vi "SI5 FPGA.vi"() -> ()   [LabVIEW 2014]
uses:
  Acquisition Engine/Acquisition Engine State.ctl
  Adapter Module Specific/Multi-Channel Analog Input Data.ctl
  <vilib>/Platform/TimedLoop/XDataNode/timing_clust.ctl
  <vilib>/Platform/TimedLoop/XDataNode/nitl_modes.ctl
  <vilib>/Platform/TimedLoop/XDataNode/wakeup.ctl
  Acquisition Engine/Acquisition Parameters.ctl
  Adapter Module Specific/Trigger Type.ctl
  <vilib>/rvi/Emulation/niFpgaSctlEmulationGetInTimedLoop.vi
  <vilib>/rvi/Emulation/niFpgaProcessEmulError.vi
  <vilib>/rvi/Emulation/niFpgaEmulationReportErrorSimple.vi
  <vilib>/rvi/Emulation/niFpgaGetClockAttributes.vi
  <vilib>/rvi/Emulation/niFpgaCriticalErrorInLSC.vi
  <vilib>/rvi/eio/common/nirviEmuTemplateMethod_errors.vi
  <vilib>/rvi/DataTransferAndStorage/Container/Common/niFpgaContainerGetUniqueNameForEmu.vi
  <vilib>/rvi/DataTransferAndStorage/Container/Common/niFpgaContainerSetEmuInfo.vi
  <vilib>/rvi/eio/common/nirviEmuReportErrorAndStop.vi
  <vilib>/rvi/DataTransferAndStorage/Container/Common/niFpgaContainerExecOnDevCompGetState.vi
  <vilib>/rvi/Emulation/niFpgaEmulationIsFPGAContextNoSignature.vi
  <vilib>/rvi/errors/niFpgaSetErrorForExecOnDevCompSimple.vi
  <vilib>/rvi/FIFO/Fifo_Resource/nirvififoEmulationSetSize.vi
  <vilib>/rvi/FIFO/Fifo_Resource/nirviFifoEmulationQueueMgr.vi
  <instcachedir>/0/nirviFifoEmulationQueueMgr_E5CAEC123FF24DC58D834DCA3CDAA9B5.lvgen/nirviFifoEmulationQueueMgr_E5CAEC123FF24DC58D834DCA3CDAA9B5_001.vi
  <vilib>/rvi/FIFO/Fifo_Resource/nirvififoEmulationDetermineInputValidOut.vi
  <vilib>/rvi/FIFO/Fifo_Resource/nirvififoEmulationCreateLock.vi
  <vilib>/rvi/FIFO/Fifo_Resource/nirvififoEmulationObtainLock.vi
  <vilib>/rvi/FIFO/Fifo_Resource/nirvififoEmulationReleaseLock.vi
  <vilib>/rvi/occurrence/nirviWaitOnOccurrenceBase.vi
  <vilib>/rvi/errors/nirviReportUnexpectedCaseInternalError.vi
  <vilib>/rvi/errors/nirviReportUnexpectedCaseInternalError (U32).vi
  <vilib>/rvi/interface/RandomDataEmulation/niFpgaRandomDataHandleErrors.vi
  <vilib>/Platform/TimedLoop/XDataNode/XDataNode.xnode
  <vilib>/eio/EIONode/EIONode.xnode
  <vilib>/rvi/LocalResourceManager/LocalResourceManager.xnode
  <vilib>/rvi/DataTransferAndStorage/Container/XNode/niFpgaContainer.xnode
  <vilib>/rvi/FIFO/Fifo_Resource/niFpgaFifoEmulationRefIn.vi
  <vilib>/Platform/TimedLoop/XDataNode/XDNodeRunTimeDep.lvlib
panel:
  in  "SPI Read":bool caption="(Mech Action: Switch)"
  in  "SPI Write":bool caption="(Mech Action: Switch)"
  in  "SPI Write Data":u16
  in  "SPI Address":u16
  in  "SPI Device Select":u8
  out "SPI Read Data":u8
  out "SPI Idle":bool
  in  "Acq Param Frames Per Stack":u16
  in  "Shutter Output":bool
  in  "Shutter Terminal Out":T1(ring)=enum.""
  out "Acq Status DC Overvoltage":bool
  in  "Acq Param Live Invert Channels":bool
  out "Acq Status Acquired Grabs":u16
  in  "Period Clock Terminal Out":T1(ring)=enum.""
  in  "Acq Trigger Terminal Out 2":T1(ring)=enum.""
  in  "Beam Clock Terminal Out 2":T1(ring)=enum.""
  in  "Frame Clock Terminal Out 2":T1(ring)=enum.""
  in  "Acq Trigger Terminal Out":T1(ring)=enum.""
  out "Debug Raw Adc Output":T2
  in  "Acq Param Live Channel Offsets":T2=[0, 0, 0, 0]
  in  "Irq Number Fifo Multi Channel Pixel Overwritten By Tag":i8=-1
  in  "Irq Number Fifo Single Channel Pixel Overwritten By Tag":i8=-1
  in  "Irq Number End of Acquisition":i8=-1
  in  "Irq Number End of Grab":i8=-1
  in  "Acq Param Grabs Per Acquisition":u16
  in  "Beam Clock Off Backward":i16
  in  "Beam Clock On Backward":i16
  in  "Beam Clock Off Forward":i16
  in  "Beam Clock On Forward":i16
  in  "Beam Clock Mode":enum8{"Trigger", "Toggle"}(ring)=enum."Toggle"
  in  "Beam Clock Terminal Out":T1(ring)=enum.""
  in  "Frame Clock Terminal Out":T1(ring)=enum.""
  in  "Stop Trigger Do Software Trig":bool
  in  "Stop Trigger Type":T3(ring)=enum."External or Software"
  in  "Stop Trigger On Falling Edge":bool
  in  "Advance Trigger Do Software Trig":bool
  in  "Advance Trigger Type":T3(ring)=enum."External or Software"
  in  "Advance Trigger On Falling Edge":bool
  in  "Stop Trigger Terminal In":T4(ring)=enum.""
  in  "Advance Trigger Terminal In":T4(ring)=enum.""
  out "Acq Status Acquired Frames":u32
  in  "Acq Param Flyback Periods":u8
  in  "Acq Param Records Per Frame":u16
  out "Adapter Module Present":bool
  in  "Acq Param Live Reverse Line Read":bool
  out "Adapter Module ID Expected":u32
  out "Adapter Module ID Inserted":u32
  in  "Acq Param Frame Tagging Enable":bool
  in  "Acq Trigger On Falling Edge":bool
  in  "Acq Trigger Type":T3(ring)=enum."External or Software"
  in  "Acq Trigger Do Software Trig":bool
  in  "Acq Trigger Terminal In":T4(ring)=enum.""
  in  "Debug Produce Dummy Data":bool
  out "Adapter Module Initialization Done":bool
  in  "Irq Number Fifo Single Channel Overflow":i8=-1
  in  "Irq Number Fifo Multi Channel Overflow":i8=-1
  in  "Irq Number End of Frame":i8=-1
  in  "Irq Fifos Data Lost Do Rearm":bool caption="(Mech Action: Latch)"
  out "Fifo Multi Channel Pixels Lost":u32
  out "Fifo Single Channel Pixels Lost":u32
  in  "Fifo Enable Multi Channel":bool
  in  "Fifo Enable Single Channel":bool
  in  "Period Clock Terminal In":T4(ring)=enum.""
  out "Adapter Module ID Mismatch":bool
  in  "Acq Param Frames Per Grab":u32 caption="Record Count"
  in  "Acq Param Live Trigger Hold Off":u16
  in  "Acq Param Samples Per Record":u16
  in  "Acq Param Live Pre Trigger Samples":u16
  in  "Period Clock On Falling Edge":bool
  out "Acq Status Acquired Records":u32
  in  "Debug Disable Raster Flip":bool
  in  "Mask Do Write Element":bool caption="(Mech Action: Latch)"
  in  "Mask Element Data":i16
  in  "Mask Write Index":i32
  out "Acq Status Acquired Pixels":u64
  in  "Adapter Module Do User Command Commit":bool caption="(Mech Action: Latch)"
  in  "Adapter Module User Command":u8
  out "Adapter Module User Command Idle":bool
  out "Adapter Module User Command Status":u8
  in  "Adapter Module User Data 0":u8
  in  "Adapter Module User Data 1":u8
  out "Adapter Module PLL Locked":bool
  in  "Acq Engine Do Reset":bool caption="(Mech Action: Latch)"
  in  "Acq Engine Do Arm":bool caption="(Mech Action: Latch)"
  in  "Period Clock Do Software Trig":bool
  in  "Acq Param Live Select Single Channel":T5(ring)
  out "Acq Status Acquired Adc Samples":u64
  out "Acq Status Engine State":T6
  in  "Period Clock Type":T3(ring)=enum."External or Software"
  # "Copyright 2014 Vidrio Technologies\nScanImage 5 software is licensed under the Apache License, Version 2.0 (the \"License\"); you may not use any files contained within the ScanImage 5 release except in compliance with the License. You may obtain a copy of the License at\n http://www.apache.org/licenses/LICENSE-2.0\nUnless required by applicable law or agreed to in writing, software distributed under the License is distributed on an \"AS IS\" BASIS, WITHOUT WARRANTIES OR CONDITIONS OF ANY KIND, either express or implied. See the License for the specific language governing permissions and limitations under the License."
  # "Acquisition Parameters"
  # "Acquisition Control"
  # "User Command Load"
  # "Fpga status"
  # "Beam Clock"
  # "SPI"
  # "Mask"
  # "Acquisition Status & Debug"
  # "Trigger I"
  # "Trigger II"
  # "Trigger III"
  # "Interrupts"
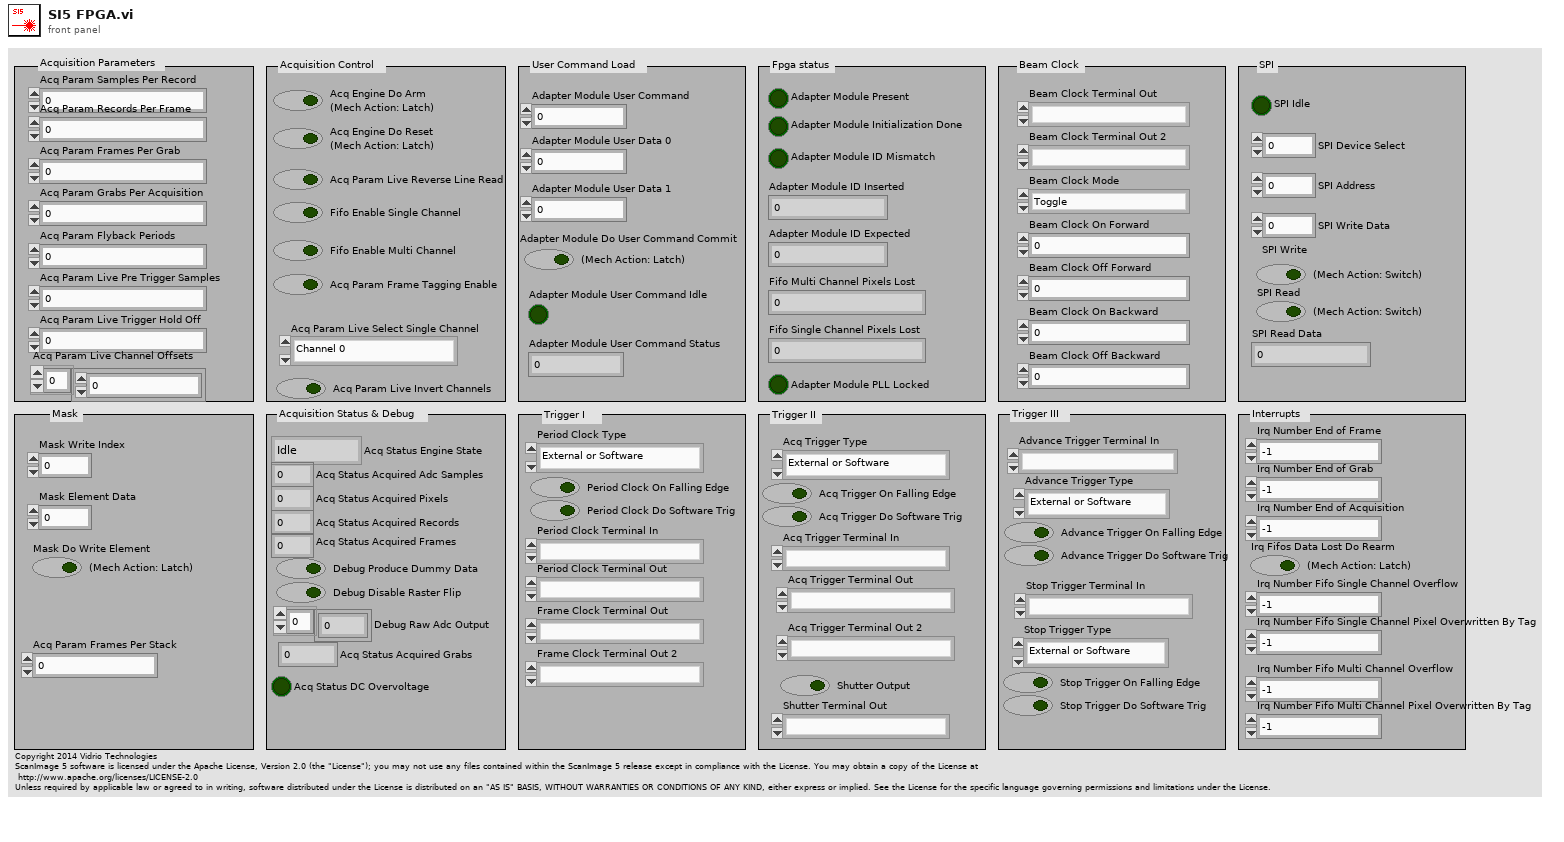
[diagram p1: front panel]
types:
  T1 = enum8{"DIO1.0", "DIO1.1", "DIO1.2", "DIO1.3", "PXI_Trig0", "PXI_Trig1", "PXI_Trig2", "PXI_Trig3", "PXI_Trig4", "PXI_Trig5", "PXI_Trig6", "PXI_Trig7", ""}
  T2 = typedef "Multi-Channel Analog Input Data.ctl" = i16[]
  T3 = enum8{"External", "Software", "Immediate", "External or Software", "None"}
  T4 = enum8{"DIO0.0", "DIO0.1", "DIO0.2", "DIO0.3", "PXI_Trig0", "PXI_Trig1", "PXI_Trig2", "PXI_Trig3", "PXI_Trig4", "PXI_Trig5", "PXI_Trig6", "PXI_Trig7", ""}
  T5 = enum8{"Channel 0", "Channel 1", "Channel 2", "Channel 3"}
  T6 = typedef "Acquisition Engine State.ctl" = enum8{"Idle", "Wait for Trigger", "Acquisition Hold Off Time", "Read Data", "Check Frame Done", "Check Grab Done", "Check Acquisition Done", "Wait Flyback Periods", "Flush Data"}
  T7 = typedef "XDNodeRunTimeDep.lvlib/timing_clust.ctl" = cluster{"Expected End [f-1]":u64, "Actual End [f-1]":u64, "Finished Late? [f-1]":bool, "Expected End [i-1]":u64, "Actual End [i-1]":u64, "Finished Late? [i-1]":bool, "Expected Start [i]":u64, "Actual Start [i]":u64, "Expected Start [f]":u64, "Actual Start [f]":u64, "Source Name":string, "Structure Name":string, "Period":i64, "Deadline":i64, "Offset":i64, "Start":i64, "Priority":i32, "Timeout":i32, "Mode":T8, "Wakeup Reason":T9, "Error":errorcluster, "Source Type":string, "Secondary Source Type":string, "Global End Time":u64, "Global Start Time":u64, "Frame Duration":u64, "Iteration Duration":u64, "Assigned CPU":i32, "I/O Scan Engine Mode":u32}
  T8 = typedef "XDNodeRunTimeDep.lvlib/nitl_modes.ctl" = enum32{"No Change", "Process missed periods, maintain original phase", "Discard missed periods, maintain original phase", "Process missed periods, ignore original phase", "Discard missed periods, ignore original phase"}
  T9 = typedef "XDNodeRunTimeDep.lvlib/wakeup.ctl" = enum32{"Normal", "Aborted", "Asynchronous wakeup", "Timing source error", "Timed loop error", "Timeout"}
  T10 = typedef "Trigger Type.ctl" = enum8{"External", "Software", "Immediate", "External or Software", "None"}
  T11 = cluster{"Acq Trigger Type":T10, "Acq Trigger On Falling Edge":bool, "Acq Software Trigger from Host":bool, "Period Clock Type":T10, "Period Clock On Falling Edge":bool, "Period Software Trigger from Host":bool, "Advance Trigger Type":T10, "Advance Trigger On Falling Edge":bool, "Advance Software Trigger from Host":bool, "Stop Trigger Type":T10, "Stop Trigger On Falling Edge":bool, "Stop Software Trigger from Host":bool}
  T12 = cluster{"Acq Engine Do Arm":bool, "Acq Engine Do Reset":bool}
  T13 = typedef "Acquisition Parameters.ctl" = cluster{"Trigger Hold Off":u16, "Samples per Record":u16, "Records Per Frame":u16, "Frames Per Grab":u32, "Grabs Per Acquisition":u16, "Flyback Periods":u8, "Frames Per Stack":u16, "Beam Clock Config":cluster{"Beam Clock Mode":enum8{"Trigger", "Toggle"}, "Beam On Forward":i16, "Beam Off Forward":i16, "Beam On Backward":i16, "Beam Off Backward":i16}}
  T14 = cluster{"Rearm FIFO Data Lost IRQs":bool, "Enable FIFO Single Channel":bool, "Enable FIFO Multi Channel":bool}
  T15 = cluster{"Bank 0":refnum<k21>, "Bank 1":refnum<k21>}
  T16 = typedef "Trigger Signals.ctl" = cluster{"Acquisition Trigger":bool, "Period Clock":bool, "Advance Trigger":bool, "Stop Trigger":bool}
  T17 = typedef "Acquisition Status.ctl" = cluster{"Reset":bool, "Start of Record":bool, "End of Record":bool, "Start of Frame":bool, "End of Frame":bool, "End of Grab":bool, "End of Acquisition":bool, "Frame Timestamp":u64, "Acq Trigger Timestamp":u64, "Next Trigger Timestamp":u64}
  T18 = typedef "Trigger Output Signals.ctl" = cluster{"Period Clock":bool, "Frame Clock":bool, "Beam Clock":bool, "Acquisition Trigger":bool}
  T19 = cluster{"Acquisition State":T6, "Updated Grabs Done":u16}
  T20 = typedef "Async Frametag Data.ctl" = cluster{"Send Frametag":bool, "End Of Grab":bool, "End of Acquisition":bool, "Next Trigger Timestamp":u64}
  T21 = cluster{"Mask Write Index":i32, "Mask Element Data":i16, "Mask Do Write Element":bool}
  T22 = cluster{"EndofLine?":bool, "Acquisition Status Out":T17}
  T23 = cluster{"Single Channel Output":cluster{"Single Channel Data out":i16, "Output Valid":bool, "Pixel Overwritten by Tag":bool}, "Multi Channel Output":cluster{"Multi Channel Data out":i16[], "Output Valid":bool, "Pixel Overwritten by Tag":bool}}
  T24 = typedef "IRQ Flags.ctl" = bool[]
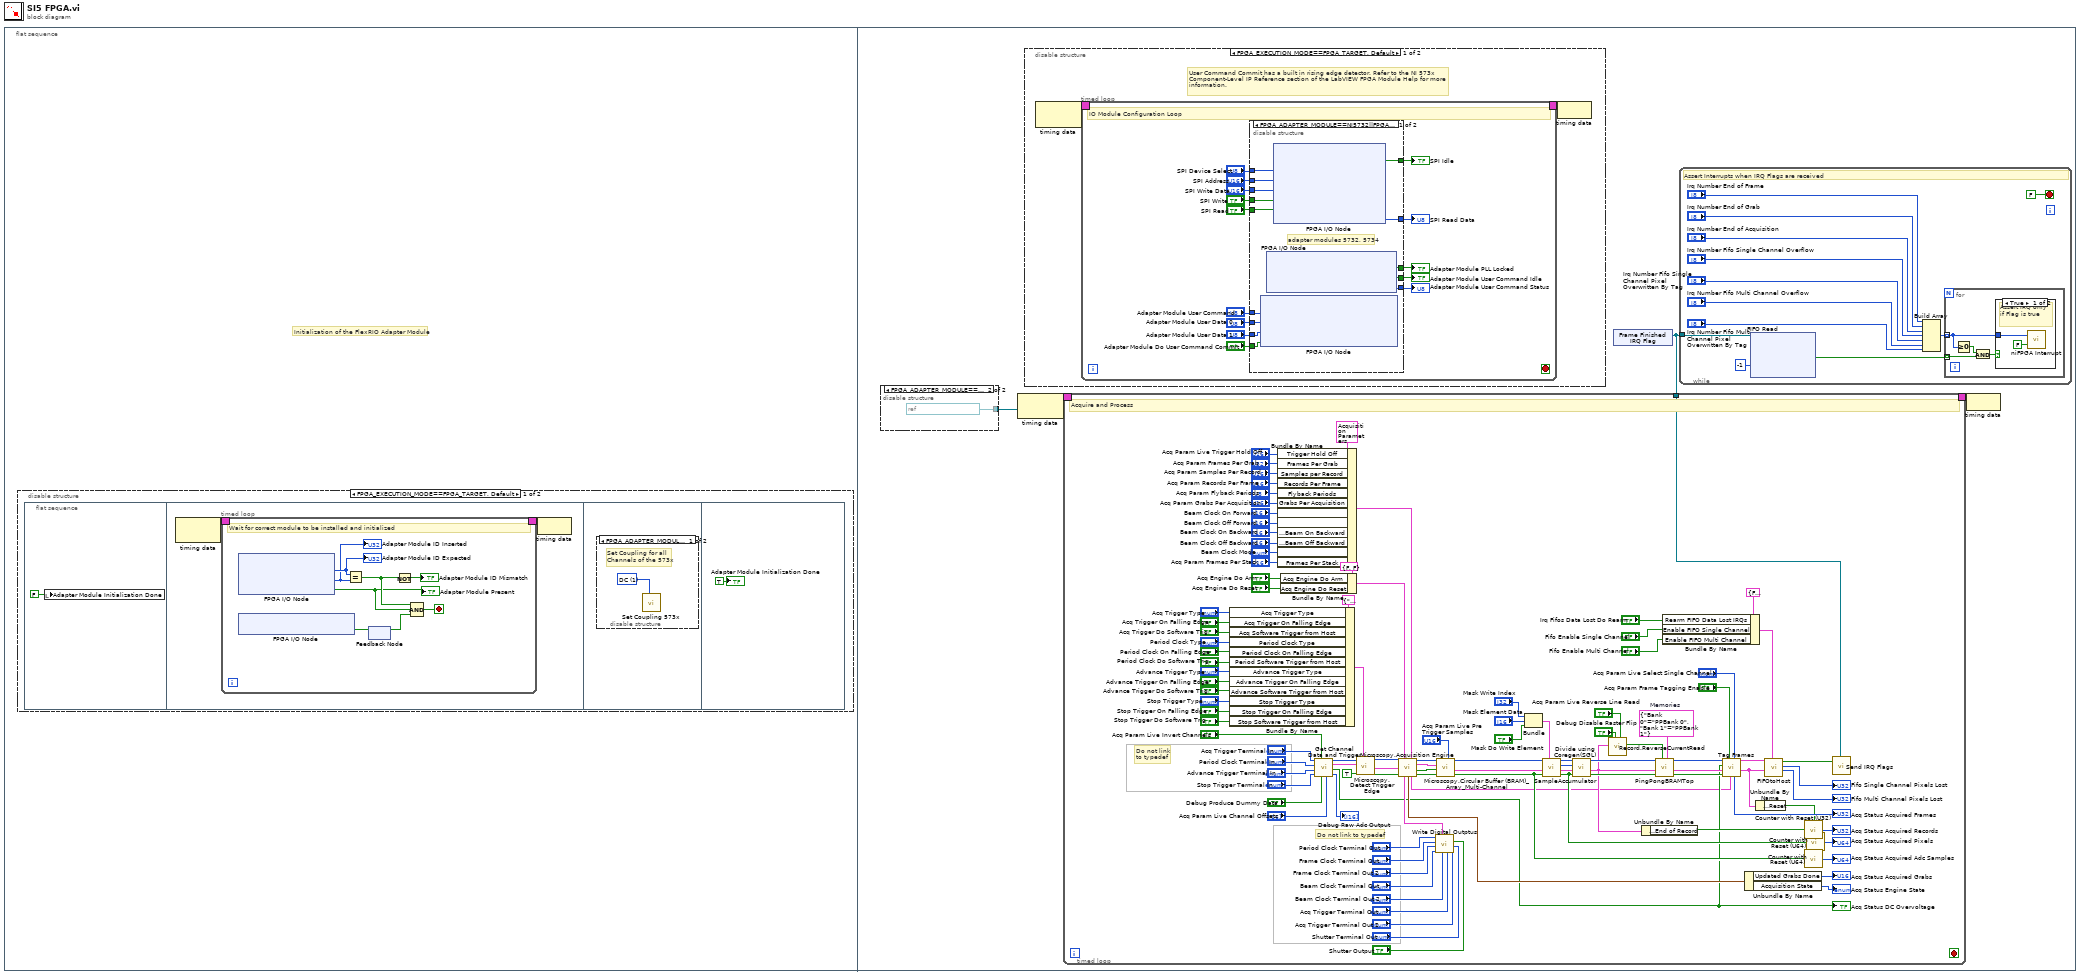
[diagram p0: block diagram]
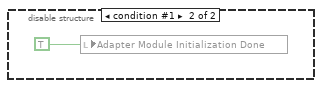
[diagram p3: hidden frame]
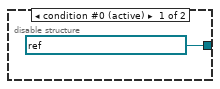
[diagram p4: hidden frame]
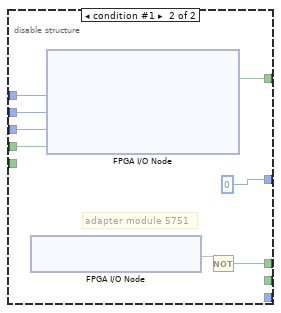
[diagram p5: hidden frame]
diagram:
  n1 = flat-sequence {
    frame #0 {
      # "Initialization of the FlexRIO Adapter Module"
      n2 = disable-structure shown="FPGA_EXECUTION_MODE==FPGA_TARGET, Default" {
        frame condition #0 (active) {
          n3 = flat-sequence {
            frame #0 {
              n4 = local write "Adapter Module Initialization Done"(FALSE ("InitializationDone")) -> ()
            }
            frame #1 {
              n5 = node-c288() -> (w3:T7)  [unwired: 1 in]
              n6 = timed-loop {
                timing: w3 -> [_]
                timing-out: [_] -> w2
                stop <- w10 stop-if-true
                # "Wait for correct module to be installed and initialized"
                n7 = xnode "FPGA I/O Node"() -> ("IO Module\\Initialization Done"=w5:bool)  [unwired: 1 in, 1 out]
                n8 = xnode "FPGA I/O Node"() -> ("Expected IO Module ID"=w11:u32, "Inserted IO Module ID"=w9:u32, "IO Module Present"=w6:bool)  [unwired: 3 in, 3 out]
                "Adapter Module ID Inserted" <- w9
                "Adapter Module ID Expected" <- w11
                "Adapter Module Present" <- w6
                n9 = Equal?(x=w11, y=w9) -> (x = y?=w7:bool)
                n10 = feedback-in #1(w5) -> ()
                n11 = feedback #1() -> (w4:bool)  [unwired: 1 in]
                n12 = Not(x=w7) -> (.not. x?=→"Adapter Module ID Mismatch":bool)
                n13 = Compound Arithmetic op=AND(w7, w6, w4) -> (w10:bool)
              }
              n14 = node-c288(w2) -> ()
            }
            frame #2 {
              n15 = disable-structure shown="FPGA_ADAPTER_MODULE==NI5732||FPGA_ADAPTER_MODULE==NI5734, Default" {
                frame condition #0 (active) {
                  w16 = u8 1 items=["DC"=1, "AC"=0] ("Coupling")
                  # "Set Coupling for all\nChannels of the 573x"
                  n16 = call "Set Coupling 573x.vi"("Coupling"=w16) -> ()  [unwired: 11 in]
                }
                frame condition #1 {
                  # "NI 5751 only supports\nDC coupling, no need\nfor additional configuration"
                }
              }
            }
            frame #3 {
              "Adapter Module Initialization Done" <- TRUE ("InitializationDone")
            }
          }
        }
        frame condition #1 {
          n17 = local write "Adapter Module Initialization Done"(TRUE ("InitializationDone")) -> ()
        }
      }
    }
    frame #1 {
      n18 = disable-structure shown="FPGA_ADAPTER_MODULE==NI5751" {
        disable-tunnel: [refnum<k21> "IO Module\\Sample Clock" ("Source Name") refnum<k21> "IO Module Clock 0" ("Source Name")] -> w19
        frame condition #0 (active) {
        }
        frame condition #1 {
        }
      }
      n19 = node-c288(w19) -> (w22:T7)
      n20 = disable-structure shown="FPGA_EXECUTION_MODE==FPGA_TARGET, Default" {
        frame condition #0 (active) {
          # "User Command Commit has a built in rising edge detector. Refer to the NI 573x Component-Level IP Reference section of the LabVIEW FPGA Module Help for more information."
          n21 = node-c288() -> (w26:T7)  [unwired: 1 in]
          n22 = timed-loop {
            timing: w26 -> [_]
            timing-out: [_] -> w25
            stop <- _ stop-if-true
            # "IO Module Configuration Loop"
            n23 = disable-structure shown="FPGA_ADAPTER_MODULE==NI5732||FPGA_ADAPTER_MODULE==NI5734, Default" {
              disable-tunnel: [w54 w61] -> w40
              disable-tunnel: [w53 _] -> w39
              disable-tunnel: [w52 _] -> w38
              disable-tunnel: "Adapter Module User Command" -> [w51 _]
              disable-tunnel: "Adapter Module User Data 0" -> [w50 _]
              disable-tunnel: "Adapter Module User Data 1" -> [w49 _]
              disable-tunnel: "Adapter Module Do User Command Commit" -> [w48 _]
              disable-tunnel: "SPI Device Select" -> [w47 w59]
              disable-tunnel: "SPI Address" -> [w46 w58]
              disable-tunnel: "SPI Write Data" -> [w45 w57]
              disable-tunnel: "SPI Write" -> [w44 w56]
              disable-tunnel: "SPI Read" -> [w43 _]
              disable-tunnel: [w42 w60] -> w28
              disable-tunnel: [w41 u8 0 ("SPI Read Data")] -> w27
              frame condition #0 (active) {
                # "adapter modules 5732, 5734"
                n24 = xnode ("FPGA I/O Node")("IO Module\\User Command"=w51, "IO Module\\User Data 0"=w50, "IO Module\\User Data 1"=w49, "IO Module\\User Command Commit"=w48) -> ()  [unwired: 4 in, 4 out]
                n25 = xnode "FPGA I/O Node"() -> ("IO Module\\PLL Locked"=w54:bool, "IO Module\\User Command Idle"=w53:bool, "IO Module\\User Command Status"=w52:u8)  [unwired: 3 in, 3 out]
                n26 = xnode "FPGA I/O Node"("IO Module\\SPI Device Select"=w47, "IO Module\\SPI Address"=w46, "IO Module\\SPI Write Data"=w45, "IO Module\\SPI Write"=w44, "IO Module\\SPI Read"=w43) -> ("IO Module\\SPI Idle"=w42:bool, "IO Module\\SPI Read Data"=w41:u8)  [unwired: 7 in, 7 out]
              }
              frame condition #1 {
                # "adapter module 5751"
                n27 = xnode "FPGA I/O Node"() -> ("IO Module\\Pll Unlocked"=w62)  [unwired: 1 in, 1 out]
                n28 = xnode "FPGA I/O Node"("IO Module\\SPI Device Select"=w59, "IO Module\\SPI Address"=w58, "IO Module\\SPI Write Data"=w57, "IO Module\\SPI Write"=w56) -> ("IO Module\\SPI Idle"=w60:bool)  [unwired: 5 in, 5 out]
                n29 = Not(x=w62) -> (.not. x?=w61:bool)
              }
            }
            "Adapter Module PLL Locked" <- w40
            "Adapter Module User Command Idle" <- w39
            "Adapter Module User Command Status" <- w38
            "SPI Idle" <- w28
            "SPI Read Data" <- w27
          }
          n30 = node-c288(w25) -> ()
        }
        frame condition #1 {
        }
      }
      n31 = xnode ("Frame Finished\nIRQ Flag")() -> ("FIFO Out"=w20:refnum<k21>)
      n32 = timed-loop {
        timing: w22 -> [_]
        timing-out: [_] -> w21
        tunnel: w20 -> [w172]
        stop <- _ stop-if-true
        w176 = T15 {"Bank 0"="PPBank 0", "Bank 1"="PPBank 1"}  # Memories
        # "Do not link to typedef"
        # "Do not link\nto typedef"
        # "Acquire and Process"
        n33 = Bundle By Name(cluster=T11 {"Acq Trigger Type"=enum."External", "Acq Trigger On Falling Edge"=FALSE, "Acq Software Trigger from Host"=FALSE, "Period Clock Type"=enum."External", "Period Clock On Falling Edge"=FALSE, "Period Software Trigger from Host"=FALSE, "Advance Trigger Type"=enum."External", "Advance Trigger On Falling Edge"=FALSE, "Advance Software Trigger from Host"=FALSE, "Stop Trigger Type"=enum."External", "Stop Trigger On Falling Edge"=FALSE, "Stop Software Trigger from Host"=FALSE} ("Trigger Configuration"), "Acq Trigger Type"="Acq Trigger Type", "Acq Trigger On Falling Edge"="Acq Trigger On Falling Edge", "Acq Software Trigger from Host"="Acq Trigger Do Software Trig", "Period Clock Type"="Period Clock Type", "Period Clock On Falling Edge"="Period Clock On Falling Edge", "Period Software Trigger from Host"="Period Clock Do Software Trig", "Advance Trigger Type"="Advance Trigger Type", "Advance Trigger On Falling Edge"="Advance Trigger On Falling Edge", "Advance Software Trigger from Host"="Advance Trigger Do Software Trig", "Stop Trigger Type"="Stop Trigger Type", "Stop Trigger On Falling Edge"="Stop Trigger On Falling Edge", "Stop Software Trigger from Host"="Stop Trigger Do Software Trig") -> (w115:T11)
        n34 = Bundle By Name(cluster=T13 {"Trigger Hold Off"=0, "Samples per Record"=0, "Records Per Frame"=0, "Frames Per Grab"=0, "Grabs Per Acquisition"=0, "Flyback Periods"=0, "Frames Per Stack"=0, "Beam Clock Config"={"Beam Clock Mode"=enum."Trigger", "Beam On Forward"=0, "Beam Off Forward"=0, "Beam On Backward"=0, "Beam Off Backward"=0}} ("Acquisition Parameters"), "Trigger Hold Off"="Acq Param Live Trigger Hold Off", "Frames Per Grab"="Acq Param Frames Per Grab", "Samples per Record"="Acq Param Samples Per Record", "Records Per Frame"="Acq Param Records Per Frame", "Flyback Periods"="Acq Param Flyback Periods", "Grabs Per Acquisition"="Acq Param Grabs Per Acquisition", "Beam Clock Config.Beam On Forward"="Beam Clock On Forward", "Beam Clock Config.Beam Off Forward"="Beam Clock Off Forward", "Beam Clock Config.Beam On Backward"="Beam Clock On Backward", "Beam Clock Config.Beam Off Backward"="Beam Clock Off Backward", "Beam Clock Config.Beam Clock Mode"="Beam Clock Mode", "Frames Per Stack"="Acq Param Frames Per Stack") -> (w143:T13)
        n35 = Bundle By Name(cluster=T12 {"Acq Engine Do Arm"=FALSE, "Acq Engine Do Reset"=FALSE}, "Acq Engine Do Arm"="Acq Engine Do Arm", "Acq Engine Do Reset"="Acq Engine Do Reset") -> (w137:T12)
        n36 = call "Get Channel Data and Trigger.vi"("Channel Offsets"="Acq Param Live Channel Offsets", "Produce Dummy Data"="Debug Produce Dummy Data", "Invert Channels"="Acq Param Live Invert Channels", "Stop Trigger Terminal"="Stop Trigger Terminal In", "Advance Trigger Terminal"="Advance Trigger Terminal In", "Period Trigger Terminal"="Period Clock Terminal In", "Acquisition Trigger Terminal"="Acq Trigger Terminal In") -> ("Raw Data"=→"Debug Raw Adc Output":T2, "Overvoltage"=w88:bool, "Trigger Signals"=w167:T16, "Data"=w184:T2)  [unwired: 1 in]
        "Acq Status DC Overvoltage" <- w88
        n37 = call "Microscopy.Detect Trigger Edge.vi"("Trigger Configuration"=w115, "Data Valid In"=TRUE, "Trigger Signals"=w167, "Analog Channel Data"=w184) -> ("Data Valid Out"=w186:bool, "Trigger Edges"=w187:T16, "Analog Channel Data"=w188:T2)  [unwired: 5 in]
        n38 = call "Microscopy.Acquisition Engine.vi"("Channel Data In"=w188, "Engine Commands"=w137, "Acquisition Parameters"=w143, "Trigger Edges"=w187, "Data Valid In"=w186) -> ("Channel Data Out"=w190:T2, "Acquisition Status"=w108:T17, "Read Data"=w139:bool, "Trigger Output Signals"=w96:T18, "Acquisition Debug Status"=w94:T19, "Async Frametag Data"=w87:T20, "Data Valid Out"=w189:bool)  [unwired: 4 in]
        n39 = call "Write Digital Outptus.vi"("Acquisition Trigger Output Terminal 2"="Acq Trigger Terminal Out 2", "Shutter Output Terminal"="Shutter Terminal Out", "Shutter Output Value"="Shutter Output", "Acquisition Trigger Output Terminal"="Acq Trigger Terminal Out", "Beam Clock Output Terminal 2"="Beam Clock Terminal Out 2", "Digital Outputs"=w96, "Beam Clock Output Terminal"="Beam Clock Terminal Out", "Frame Clock Ouput Terminal 2"="Frame Clock Terminal Out 2", "Frame Clock Ouput Terminal"="Frame Clock Terminal Out", "Period Clock Ouput Terminal"="Period Clock Terminal Out") -> ()  [unwired: 2 in]
        n40 = call "Microscopy.Circular Buffer (BRAM)_Array_Multi-Channel.vi"("Input Write Data"=w190, "Acquisition Status In"=w108, "Read Data?"=w139, "Input Valid"=w189, "Acq Param Pre Trigger Samples"="Acq Param Live Pre Trigger Samples") -> ("Output Write Data"=w142:T2, "Acquisition Status Out"=w141:T17, "Output Valid"=w140:bool)  [unwired: 3 in]
        n41 = Bundle("Mask Write Index"="Mask Write Index", "Mask Element Data"="Mask Element Data", "Mask Do Write Element"="Mask Do Write Element") -> (w158:T21)  [unwired: 1 in]
        n42 = call "SampleAccumulator.vi"("Write Element Data"=w158, "Input Valid"=w140, "Acquisition Status In"=w141, "Input Data"=w142) -> ("End of Acc?"=w169:bool, "Line Status Out"=w180:T22, "Final Count"=w182:i16, "Accumulated Value"=w178:i32[])  [unwired: 3 in, 1 out]
        n43 = call "Divide using Coregen(SGL).vi"("Input Valid"=w169, "Line Status In"=w180, "Divisor"=w182, "Dividend"=w178) -> ("Output Valid"=w181:bool, "Line Status Out"=w131:T22, "All Channel Data"=w177:T2)  [unwired: 4 in, 1 out]
        n44 = call "Record.ReverseCurrentRead.vi"("Reverse Read"="Acq Param Live Reverse Line Read", "DisableRasterFlip"="Debug Disable Raster Flip", "Line Status In"=w131) -> ("Reverse Read"=w171:bool)  [unwired: 8 in]
        n45 = Unbundle By Name(w131) -> ("Acquisition Status Out.End of Record"=w150:bool)
        n46 = call "PingPongBRAMTop.vi"("Memories"=w176, "ReverseLineRead?"=w171, "Input Valid"=w181, "Line Status In"=w131, "Data In"=w177) -> ("Output Valid"=w156:bool, "Line Status Out"=w130:T22, "Data Out"=w157:i16[])  [unwired: 4 in]
        n47 = Bundle By Name(cluster=T14 {"Rearm FIFO Data Lost IRQs"=FALSE, "Enable FIFO Single Channel"=FALSE, "Enable FIFO Multi Channel"=FALSE} ("FIFO control"), "Rearm FIFO Data Lost IRQs"="Irq Fifos Data Lost Do Rearm", "Enable FIFO Single Channel"="Fifo Enable Single Channel", "Enable FIFO Multi Channel"="Fifo Enable Multi Channel") -> (w146:T14)
        n48 = call "Tag Frames.vi"("Single Channel Select"="Acq Param Live Select Single Channel", "Frame Tag Bypass"=w87, "Enable Frame Tagging"="Acq Param Frame Tagging Enable", "Input Valid"=w156, "Line Status In"=w130, "DC Overvoltage"=w88, "Data In"=w157) -> ("Line Status Out"=w106:T22, "Data"=w154:T23, "Frames Acquired"=→"Acq Status Acquired Frames":u32)  [unwired: 2 in]
        n49 = Unbundle By Name(w94) -> ("Updated Grabs Done"=→"Acq Status Acquired Grabs":u16, "Acquisition State"=→"Acq Status Engine State":T6)
        n50 = Unbundle By Name(w106) -> ("Acquisition Status Out.Reset"=w107:bool)
        n51 = call "FIFOtoHost.vi"("FIFO control"=w146, "Line Status In"=w106, "Data"=w154) -> ("FIFO Multi Channels Pixels Lost"=→"Fifo Multi Channel Pixels Lost":u32, "FIFO Single Channels Pixels Lost"=→"Fifo Single Channel Pixels Lost":u32, "IRQ Flags Out"=w151:T24)  [unwired: 6 in]
        n52 = call "Counter with Reset (U32).vi"("Reset?"=w107, "Increment"=w150) -> ("Counter"=→"Acq Status Acquired Records":u32)  [unwired: 13 in]
        n53 = call "Counter with Reset (U64).vi"("Reset?"=w107, "Increment"=w140) -> ("Counter"=→"Acq Status Acquired Adc Samples":u64)  [unwired: 13 in]
        n54 = call "Counter with Reset (U64).vi"("Reset?"=w107, "Increment"=w169) -> ("Counter"=→"Acq Status Acquired Pixels":u64)  [unwired: 13 in]
        n55 = call "Send IRQ Flags.vi"("IRQ Flag FIFO"=w172, "IRQ Flags In"=w151) -> ()  [unwired: 10 in]
      }
      n56 = while {
        tunnel: w20 -> [w77]
        stop <- FALSE stop-if-true
        # "Assert Interrupts when IRQ Flags are received"
        n57 = xnode ("FIFO Read")("Timeout"=-1, "FIFO In"=w77) -> ("Element"=w73:bool[])  [unwired: 2 out]
        n58 = Build Array("Irq Number End of Frame", "Irq Number End of Grab", "Irq Number End of Acquisition", "Irq Number Fifo Single Channel Overflow", "Irq Number Fifo Single Channel Pixel Overwritten By Tag", "Irq Number Fifo Multi Channel Overflow", "Irq Number Fifo Multi Channel Pixel Overwritten By Tag") -> (w72:i8[])
        n59 = for {
          tunnel: w73 -> [w79] mode=indexing
          tunnel: w72 -> [w82] mode=indexing
          n60 = Greater Or Equal To 0?(x=w82) -> (x >= 0?=w81:bool)
          n61 = And(x=w81, y=w79) -> (x .and. y?=w80:bool)
          n62 = case shown="True" w80 {
            tunnel: w82 -> [w84 _]
            frame True {
              # "Assert IRQ only\nif Flag is true"
              n63 = call <vilib>:"niFPGA Interrupt.vi"("Wait Until Cleared (F)"=FALSE, "IRQ Number (0)"=w84) -> ()  [unwired: 1 in]
            }
            frame False {
            }
          }
        }
      }
      n64 = node-c288(w21) -> ()
    }
  }
